vi "LightingLab.vi"() -> ()   [LabVIEW 2014]
panel:
  out "Indicator Light":bool
  in  "Master":bool
  in  "Switch C":bool
  in  "Switch D":bool
  in  "Switch B":bool
  in  "Switch A":bool
  out "Light D":bool
  out "LIght C":bool
  out "Light B":bool
  out "Light A":bool
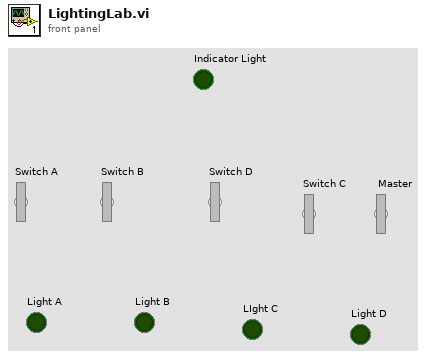
[diagram p1: front panel]
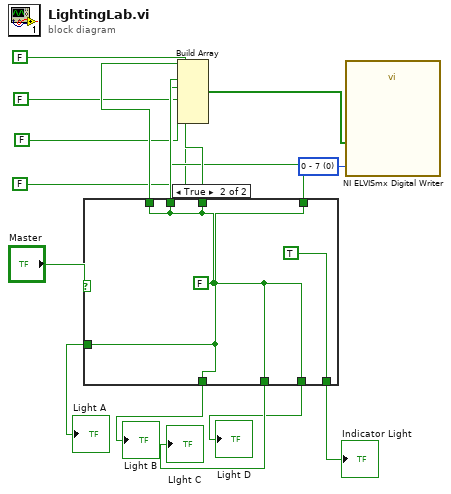
[diagram p0: block diagram]
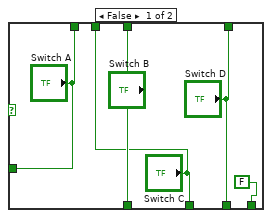
[diagram p2: hidden frame]
diagram:
  w1 = u16 0 items=["0 - 7", "8 - 15", "16 - 23"] ("Lines to Write")
  n1 = case shown="True" "Master" {
    tunnel: ["Switch A" w22] -> w16
    tunnel: ["Switch B" w22] -> w15
    tunnel: ["Switch C" w22] -> w14
    tunnel: ["Switch D" w22] -> w13
    tunnel: [FALSE TRUE] -> w12
    tunnel: ["Switch A" w22] -> w11
    tunnel: ["Switch B" w22] -> w10
    tunnel: ["Switch C" w22] -> w9
    tunnel: ["Switch D" w22] -> w8
    frame False {
    }
    frame True {
      w22 = FALSE
    }
  }
  "Light A" <- w16
  "Light B" <- w15
  "LIght C" <- w14
  "Light D" <- w13
  "Indicator Light" <- w12
  n2 = Build Array(w11, w10, w9, w8, FALSE, FALSE, FALSE, FALSE) -> (w2:bool[])
  n3 = call "NI ELVISmx Digital Writer"("Lines to Write"=w1, "DO Lines"=w2) -> ()  [unwired: 17 in, 1 out]
